vi "Get Type.vi"(8 "error in (no error)":errorcluster, 11 "I8 Connection in":refnum<class "I8 Connection.lvclass">) -> (0 "error out":errorcluster, 2 "Type":T1, 3 "I8 Connection out":refnum<class "I8 Connection.lvclass">)   [LabVIEW 2020, in "Parallel Block.lvlib" / "I8 Connection.lvclass"]
uses:
  I8 Connection.lvclass
  I8 Connection.lvclass/I8 Connection.ctl
  Value Type.ctl
  Parallel Block.lvlib
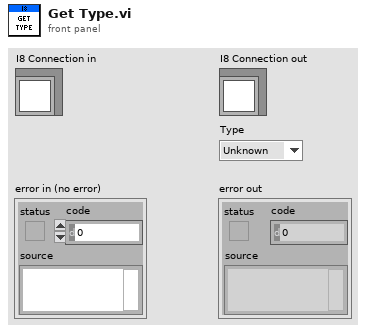
[diagram p1: front panel]
types:
  T1 = typedef "Parallel Block.lvlib/Value Type.ctl" = enum16{"Unknown", "Bool", "U8", "U16", "U32", "U64", "I8", "I16", "I32", "I64", "SGL", "DBL", "CSG", "CDB", "CDBWfm", "String", "DBLWfm"}
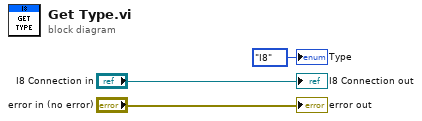
[diagram p0: block diagram]
diagram:
  "error out" <- "error in (no error)"
  "I8 Connection out" <- "I8 Connection in"
  "Type" <- Value_Type."I8" ("Type")
